vi "stack_dupn.vi"(8 "error in (no error)":errorcluster, 10 "n":i32=1, 11 "Lua in":refnum<class "Lua.lvclass">) -> (0 "error out":errorcluster, 3 "Lua out":refnum<class "Lua.lvclass">)   [LabVIEW 2020, in "Lua for LabVIEW.lvlib" / "Lua.lvclass"]
doc: "Rotates the stack elements between the valid index idx and the top of the stack. The elements are rotated n positions in the direction of the top, for a positive n, or -n positions in the direction of the bottom, for a negative n. The absolute value of n must not be greater than the size of the slice being rotated. This function cannot be called with a pseudo-index, because a pseudo-index is not an actual stack position."
uses:
  Lua.lvclass
  Lua.lvclass/Lua.ctl
  lib/lua.dll/lua.dll.lvlib
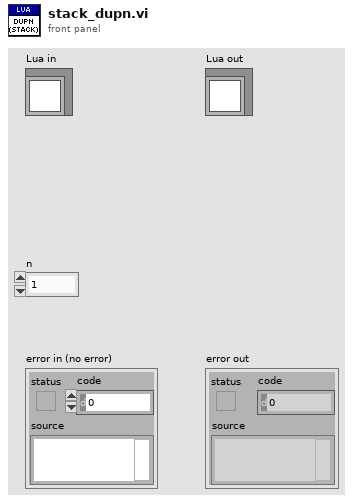
[diagram p1: front panel]
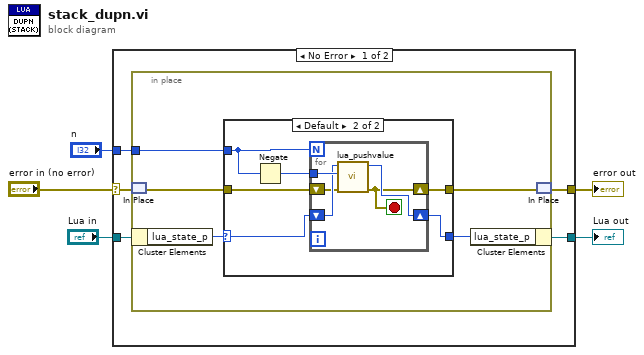
[diagram p0: block diagram]
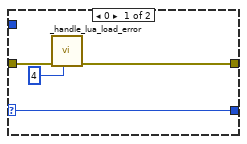
[diagram p2: hidden frame]
diagram:
  n1 = case shown="No Error" "error in (no error)" {
    selector: "error in (no error)" -> [w7 w32]
    tunnel: [w8 w32] -> w4
    tunnel: [w9 w31] -> w2
    tunnel: "Lua in" -> [w10 w31]
    tunnel: "n" -> [w6 _]
    frame No Error {
      n2 = in-place {
        in-place-border: w6 -> [w11]
        n3 = in-place-match #1(w7) -> (w13:errorcluster)
        n4 = in-place-cluster #2(w10) -> ("lua_state_p"=w14:u64)
        n5 = case shown="Default" w14 {
          selector: w14 -> [w19 w22]
          tunnel: [w19 w21] -> w15
          tunnel: w13 -> [w16 w25]
          tunnel: [w17 w20] -> w12
          tunnel: w11 -> [_ w24]
          frame 0 {
            n6 = call "_handle_lua_load_error.vi"("lua_load errcode"=4, "error in (no error)"=w16) -> ("error out"=w17:errorcluster)  [unwired: 9 in]
          }
          frame Default {
            n7 = Negate(x=w24) -> (-x=w23:i32)
            n8 = for {
              N: w24 -> [_]
              shift-right: [w28] -> w21
              shift-left: w22 -> [w29]
              shift-right: [w26] -> w20
              shift-left: w25 -> [w27]
              tunnel: w23 -> [w30]
              stop <- w26 stop-if-true
              n9 = call "lua_pushvalue.vi"("error in (no error)"=w27, "index"=w30, "lua_state_p"=w29) -> ("error out"=w26:errorcluster, "lua_state_p out"=w28:u64)  [unwired: 7 in]
            }
          }
        }
        n10 = in-place-cluster #2("lua_state_p"=w15) -> (w9:refnum<class "Lua.lvclass">)
        n11 = in-place-match #1(w12) -> (w8:errorcluster)
      }
    }
    frame Error {
    }
  }
  "error out" <- w4
  "Lua out" <- w2
